vi "CLC_Gen3_L1_eleGainPhase_ENA.vi"() -> ()   [LabVIEW 2023, in "Clover_Cell.lvlib"]
uses:
  lib/CTL/Keysight_VNA.ctl
  Clover_Cell.lvlib
  lib/Keysight/Keysight.lvlib
panel:
  in  "Waiting Time(ms)":u32=100
  in  "sParameter":i32=21
  in  "Step_Freq(GHz)":dbl=0.5 format="%#_13g"
  in  "Stop_Freq(GHz)":dbl=31.5
  in  "Start_Freq(GHz)":dbl=26.5
  in  "Polarity":u16(ring) items=["H", "V"]
  in  "TRXmode":u16(ring)=1 items=["Rx"=2, "Tx"=1]
  out "Step-2":bool
  out "PHASE 2":i32
  out "GAIN 2":i32
  out "Channel 2":i32
  out "Step-1":bool
  out "Channel":i32
  out "GAIN":i32
  out "PHASE":i32
  out "Marker_array":dbl[](array[numeric])
  out "Phase":dbl[][](graph)
  in  "FileName_Note":string
  in  "VISA resource name":refnum<visa-resource-name>="TCPIP0::192.168.100.12::inst0::INSTR"
  out "Return State":bool
  out "output cluster":T1={"address"="192.168.100.111", "remote port or service name"=5025, "timeout ms (60000)"=10000}
  out "Gain":dbl[][](graph)
  out "error out":errorcluster
  # "CLC-Gen3-L1-eleGainPhase-Sweep-ENA"
  # "Setting"
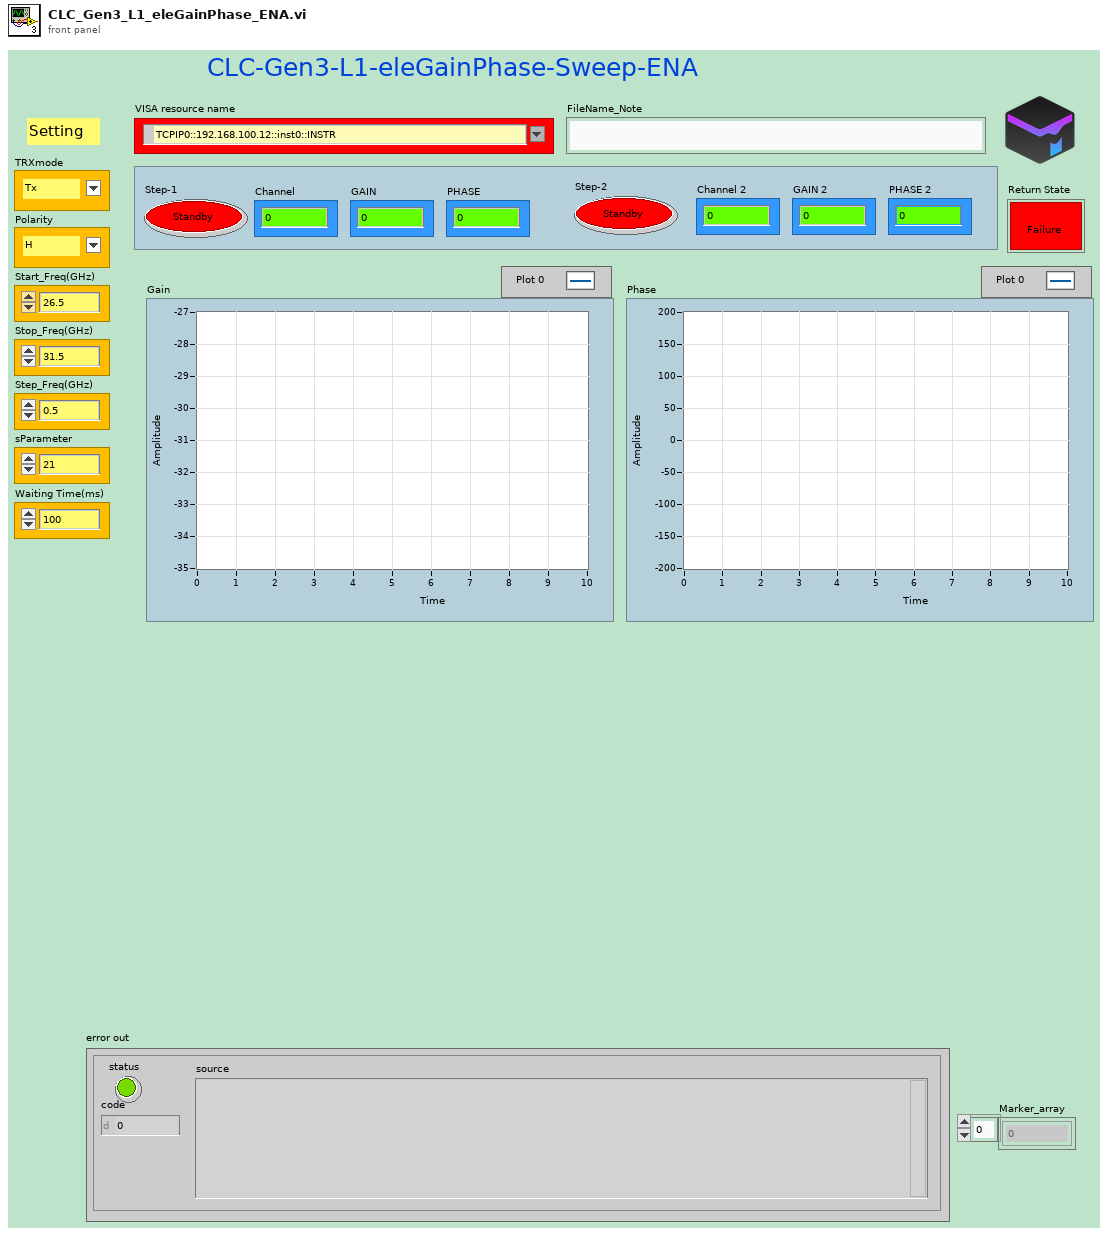
[diagram p1: front panel]
types:
  T1 = cluster{"address":string, "remote port or service name":u16, "timeout ms (60000)":i32}
  T2 = typedef "Keysight_VNA.ctl" = enum16{"Init", "queryMarker", "setSweepPoint", "setMarkerFreq", "setMeasureFormat", "setFreqStartStop", "setMarkerOnOFF", "setMarkerFormat_LOGP", "setMeasPAR_S", "setTriggerSingle", "Trigger_Save_SnP", "Trigger_Single", "Close"}
  T3 = cluster{"Mode":u16, "Polarity":u16, "CH_ON/OFF":u16, "Channel":i32, "Gain":i32, "Phase":i32}
  T4 = cluster{"setSweepPoint":i32, "Meas":i32, "Mark":i32, "Freq_GHz":dbl, "Start_Freq(GHz)":dbl, "Stop_Freq(GHz)":dbl, "sParameter":i32}
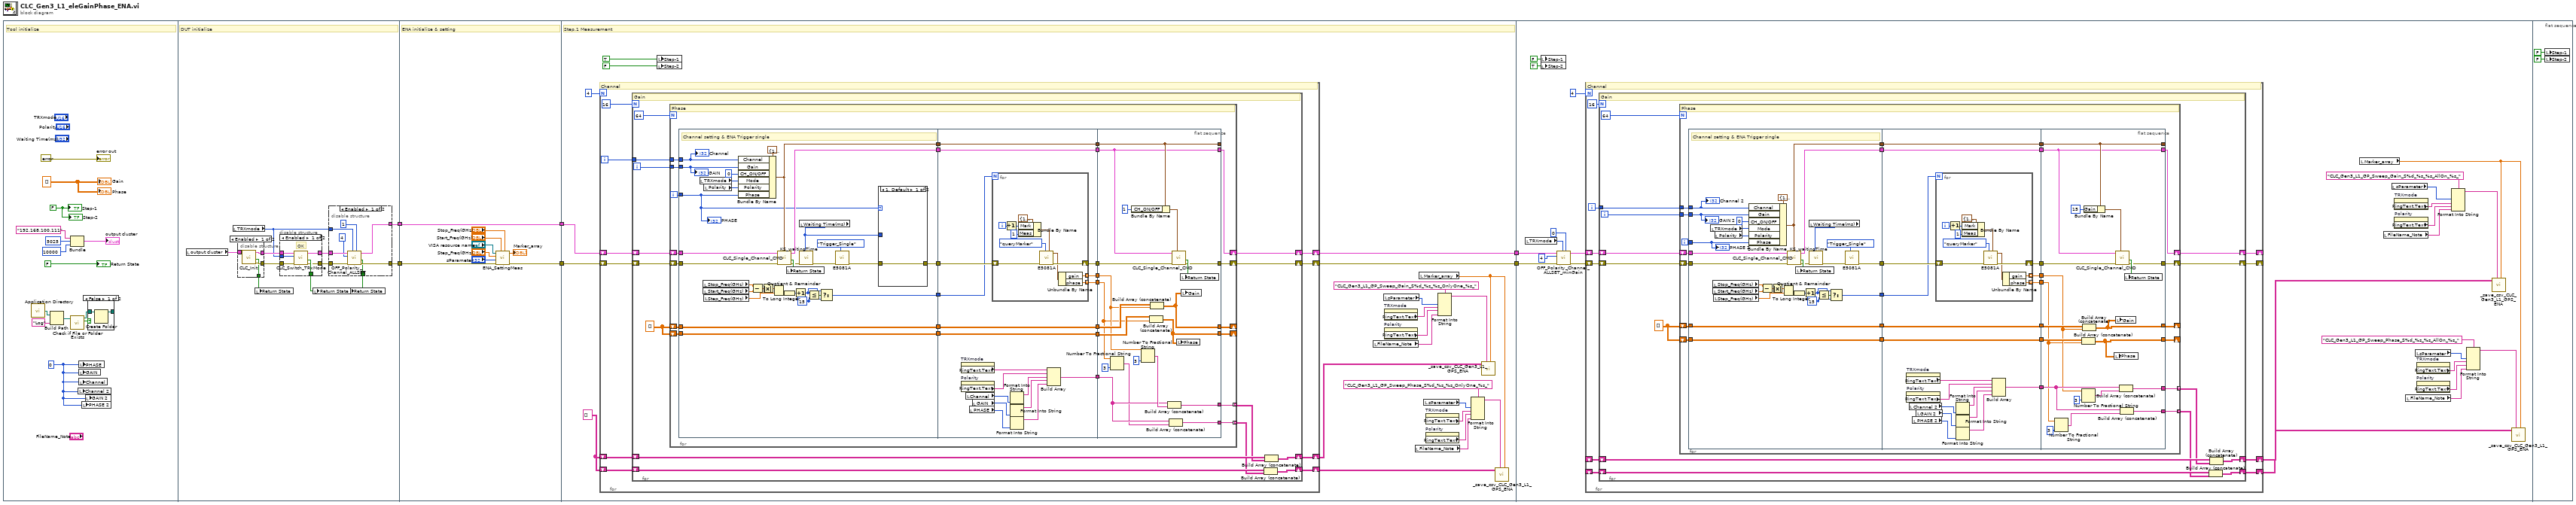
[diagram p0: block diagram]
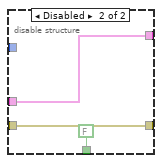
[diagram p3: hidden frame]
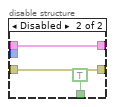
[diagram p4: hidden frame]
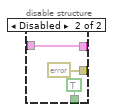
[diagram p5: hidden frame]
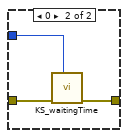
[diagram p6: hidden frame]
diagram:
  n1 = flat-sequence {
    tunnel: [w25] -> w6
    tunnel: [w29] -> w5
    tunnel: w6 -> [w70]
    tunnel: w5 -> [w63]
    tunnel: [w70] -> w4
    tunnel: [w64] -> w3
    tunnel: w4 -> [w93]
    tunnel: w3 -> [w90]
    tunnel: [w92] -> w2
    tunnel: [w91] -> w1
    tunnel: w2 -> [w249]
    tunnel: w1 -> [w250]
    frame #0 {
      w8 = FALSE ("Step-1")
      w7 = 0 ("PHASE")
      w9 = dbl[][] []
      # "Tool initialize"
      n2 = call <vilib>:"Application Directory.vi"() -> ("Application Directory"=w13:path)
      n3 = Build Path(base path=w13, name or relative path="Log") -> (appended path=w10:path)
      n4 = Bundle("address"="192.168.100.111", "remote port or service name"=u16 5025, "timeout ms (60000)"=10000) -> (→"output cluster":T1)  [unwired: 1 in]
      n5 = call <vilib>:"Check if File or Folder Exists.vi"("path"=w10) -> ("file or folder exists?"=w12:bool, "dup path"=w11:path)  [unwired: 8 in, 1 out]
      n6 = local write "Channel 2"(w7) -> ()
      n7 = local write "PHASE"(w7) -> ()
      n8 = local write "GAIN"(w7) -> ()
      n9 = local write "Channel"(w7) -> ()
      n10 = local write "PHASE 2"(w7) -> ()
      n11 = local write "GAIN 2"(w7) -> ()
      n12 = case shown="False" w12 {
        tunnel: w11 -> [w22 w23]
        tunnel: [w21 w23] -> _
        frame False {
          n13 = Create Folder(path (use dialog)=w22) -> (created path=w21:path)  [unwired: 2 in, 2 out]
        }
        frame True {
        }
      }
      "error out" <- errorcluster {"status"=FALSE, "code"=0, "source"=""} ("error out")
      "Return State" <- FALSE ("OK?")
      "Gain" <- w9
      "Phase" <- w9
      "Step-1" <- w8
      "Step-2" <- w8
    }
    frame #1 {
      # "DUT initialize"
      n14 = local read "output cluster"() -> (w34:T1)
      n15 = local read "TRXmode"() -> (w24:u16)
      n16 = disable-structure shown="Enabled" {
        disable-tunnel: w34 -> [w58 w61]
        disable-tunnel: [w57 w61] -> w33
        disable-tunnel: [w56 errorcluster {"status"=FALSE, "code"=0, "source"=""} ("error in (no error)")] -> w31
        disable-tunnel: [w55 TRUE ("OK?")] -> w26
        frame Enabled {
          n17 = call "CLC_Init.vi"("TCPIPin"=w58) -> ("error out"=w56:errorcluster, "Status"=w55:bool, "TCPIPin 2"=w57:T1)  [unwired: 8 in]
        }
        frame Disabled {
        }
      }
      n18 = local write "Return State"(w26) -> ()
      n19 = disable-structure shown="Enabled" {
        disable-tunnel: w33 -> [w51 w53]
        disable-tunnel: [w50 TRUE ("OK?")] -> w32
        disable-tunnel: w31 -> [w49 w52]
        disable-tunnel: [w48 w52] -> w30
        disable-tunnel: [w47 w53] -> w28
        disable-tunnel: w24 -> [w46 _]
        frame Enabled {
          # "OK"
          n20 = call "CLC_Switch_TRxMode.vi"("error in (no error)"=w49, "Text Ring"=w46, "TCPIPin"=w51) -> ("error out"=w48:errorcluster, "OK?"=w50:bool, "TCPIPin 2"=w47:T1)  [unwired: 6 in]
        }
        frame Disabled {
        }
      }
      n21 = local write "Return State"(w32) -> ()
      n22 = disable-structure shown="Enabled" {
        disable-tunnel: w30 -> [w42 w44]
        disable-tunnel: [w41 w44] -> w29
        disable-tunnel: w28 -> [w40 w43]
        disable-tunnel: [w39 FALSE ("OK?")] -> w27
        disable-tunnel: w24 -> [w37 _]
        disable-tunnel: [w35 w43] -> w25
        frame Enabled {
          n23 = call "OFF_Polarity_Channel_ALLSET.vi"("CH_ON:0/OFF:1"=u16 1, "Mode"=w37, "error in"=w42, "Channel"=4, "TCPIPin"=w40) -> ("error out"=w41:errorcluster, "OK?"=w39:bool, "TCPIPout"=w35:T1)  [unwired: 4 in]
        }
        frame Disabled {
        }
      }
      n24 = local write "Return State"(w27) -> ()
    }
    frame #2 {
      # "ENA initialize & setting"
      n25 = call "ENA_SettingMeas.vi"("Stop_Freq(GHz)"="Stop_Freq(GHz)", "Start_Freq(GHz)"="Start_Freq(GHz)", "error in"=w63, "sParameter"="sParameter", "Step_Freq(GHz)"="Step_Freq(GHz)", "VISA IN"="VISA resource name") -> ("error out"=w64:errorcluster, "Marker_array"=→"Marker_array":dbl[])  [unwired: 4 in]
    }
    frame #3 {
      w88 = string[][] []
      # "Step.1 Measurement"
      n26 = for {
        N: 4 -> [_]
        shift-right: [w102] -> w92
        shift-left: w93 -> [w103]
        shift-right: [w101] -> w91
        shift-left: w90 -> [w100]
        shift-right: [w95] -> w87
        shift-left: w88 -> [w97]
        shift-right: [w94] -> w86
        shift-left: w88 -> [w96]
        i -> [w98]
        # "Channel"
        n27 = for {
          N: 16 -> [_]
          shift-right: [w116] -> w102
          shift-left: w103 -> [w117]
          shift-right: [w115] -> w101
          shift-left: w100 -> [w114]
          tunnel: w98 -> [w112]
          shift-right: [w106] -> w95
          shift-left: w97 -> [w110]
          shift-right: [w105] -> w94
          shift-left: w96 -> [w109]
          i -> [w111]
          w104 = dbl[][] []
          # "Gain"
          n28 = for {
            N: 64 -> [_]
            shift-right: [w132] -> w116
            shift-left: w117 -> [w144]
            shift-right: [w131] -> w115
            shift-left: w114 -> [w143]
            tunnel: w112 -> [w142]
            tunnel: w111 -> [w141]
            tunnel: [w127] -> w108 mode=indexing
            tunnel: [w126] -> w107 mode=indexing
            shift-right: [w119] -> _
            shift-left: w104 -> [w123]
            shift-right: [w118] -> _
            shift-left: w104 -> [w120]
            i -> [w140]
            # "Phase"
            n29 = flat-sequence {
              tunnel: w144 -> [w173]
              tunnel: w143 -> [w172]
              tunnel: w142 -> [w171]
              tunnel: w141 -> [w168]
              tunnel: w140 -> [w145]
              tunnel: [w147] -> w139
              tunnel: [w153] -> w138
              tunnel: [w152] -> w137
              tunnel: [w151] -> w136
              tunnel: [w150] -> w124
              tunnel: w123 -> [w150]
              tunnel: [w149] -> w121
              tunnel: w120 -> [w149]
              tunnel: w139 -> [w196]
              tunnel: w138 -> [w195]
              tunnel: w137 -> [w194]
              tunnel: w136 -> [w193]
              tunnel: [w197] -> w135
              tunnel: [w195] -> w134
              tunnel: [w194] -> w133
              tunnel: [w192] -> w130
              tunnel: [w191] -> w129
              tunnel: [w182] -> w128
              tunnel: [w181] -> w125
              tunnel: w124 -> [w181]
              tunnel: [w180] -> w122
              tunnel: w121 -> [w180]
              tunnel: [w225] -> _
              tunnel: [w222] -> w132
              tunnel: [w227] -> w131
              tunnel: w135 -> [w226]
              tunnel: w134 -> [w222]
              tunnel: w133 -> [w225]
              tunnel: w130 -> [w212]
              tunnel: w129 -> [w211]
              tunnel: w128 -> [w218]
              tunnel: [w216] -> w127
              tunnel: [w215] -> w126
              tunnel: w125 -> [w214]
              tunnel: w122 -> [w213]
              tunnel: [w210] -> w119
              tunnel: [w209] -> w118
              frame #0 {
                w163 = 15 ("y")
                # "Channel setting & ENA Trigger single"
                n30 = local read "TRXmode"() -> (w169:u16)
                n31 = local read "Stop_Freq(GHz)"() -> (w156:dbl)
                n32 = local read "Start_Freq(GHz)"() -> (w155:dbl)
                n33 = local read "Step_Freq(GHz)"() -> (w154:dbl)
                n34 = local read "Polarity"() -> (w170:u16)
                n35 = Bundle By Name(cluster=T3 {"Mode"=1, "Polarity"=1, "CH_ON/OFF"=1, "Channel"=0, "Gain"=0, "Phase"=0} ("Channel params"), "Channel"=w171, "Gain"=w168, "CH_ON/OFF"=u16 0, "Mode"=w169, "Polarity"=w170, "Phase"=w145) -> (w152:T3)
                n36 = Subtract(x=w156, y=w155) -> (x-y=w162:dbl)
                n37 = Absolute Value(x=w162) -> (abs(x)=w161:dbl)
                n38 = Quotient & Remainder(x=w161, y=w154) -> (floor(x/y)=w160:dbl)  [unwired: 1 out]
                n39 = call "CLC_Single_Channel_CMD.vi"("Channel params"=w152, "error in"=w172, "TCPIPin"=w173) -> ("error out"=w167:errorcluster, "OK?"=w174:bool, "TCPIPout"=w153:T1)  [unwired: 6 in]
                n40 = To Long Integer(number=w160) -> (32bit integer=w159:i32)
                n41 = local write "Return State"(w174) -> ()
                n42 = Increment(x=w159) -> (x+1=w157:i32)
                n43 = local read "Waiting Time(ms)"() -> (w146:u32)
                n44 = call "KS_waitingTime.vi"("Waiting Time(ms)"=w146, "error in"=w167) -> ("error out"=w165:errorcluster)  [unwired: 9 in]
                n45 = Less Or Equal?(x=w157, y=w163) -> (x <= y?=w158:bool)
                n46 = Select(t=w157, s=w158, f=w163) -> (s? t:f=w151:i32)
                n47 = call "E5081A.vi"("Function_VNA"=Keysight_VNA."Trigger_Single", "error in"=w165) -> ("error out"=w148:errorcluster)  [unwired: 8 in, 1 out]
                n48 = case shown="1, Default" w145 {
                  tunnel: w148 -> [w176 w179]
                  tunnel: [w176 w178] -> w147
                  tunnel: w146 -> [_ w177]
                  frame 1, Default {
                  }
                  frame 0 {
                    n49 = call "KS_waitingTime.vi"("Waiting Time(ms)"=w177, "error in"=w179) -> ("error out"=w178:errorcluster)  [unwired: 9 in]
                  }
                }
                "PHASE" <- w145
                "GAIN" <- w168
                "Channel" <- w171
              }
              frame #1 {
                n50 = property on="TRXmode" class="Ring (strict)"() -> ("RingText.Text"=w187:string)  [unwired: 2 in, 2 out]
                n51 = property on="Polarity" class="Ring (strict)"() -> ("RingText.Text"=w186:string)  [unwired: 2 in, 2 out]
                n52 = local read "Channel"() -> (w190:i32)
                n53 = local read "PHASE"() -> (w188:i32)
                n54 = local read "GAIN"() -> (w189:i32)
                n55 = for {
                  N: w193 -> [_]
                  shift-right: [w207] -> w197
                  shift-left: w196 -> [w208]
                  tunnel: [w199] -> w192 mode=indexing
                  tunnel: [w198] -> w191 mode=indexing
                  i -> [w204]
                  n56 = Increment(x=w204) -> (x+1=w202:i32)
                  n57 = Bundle By Name(cluster=T4 {"setSweepPoint"=11, "Meas"=1, "Mark"=0, "Freq_GHz"=0.0, "Start_Freq(GHz)"=0.0, "Stop_Freq(GHz)"=0.0, "sParameter"=1} ("Input"), "Mark"=w202, "Meas"=1) -> (w201:T4)
                  n58 = call "E5081A.vi"("Input"=w201, "Function_VNA"=Keysight_VNA."queryMarker", "error in"=w208) -> ("error out"=w207:errorcluster, "queryMarker"=w200:cluster{"gain":dbl, "phase":dbl})  [unwired: 7 in]
                  n59 = Unbundle By Name(w200) -> ("gain"=w199:dbl, "phase"=w198:dbl)
                }
                n60 = Format Into String(w190) -> (resulting string=w185:string)  [unwired: 3 in, 1 out]
                n61 = Format Into String(w189) -> (resulting string=w184:string)  [unwired: 3 in, 1 out]
                n62 = Format Into String(w188) -> (resulting string=w183:string)  [unwired: 3 in, 1 out]
                n63 = Build Array(w187, w186, w185, w184, w183) -> (w182:string[])
              }
              frame #2 {
                n64 = Number To Fractional String(number=w211, precision (6)=i16 3) -> (F-format string=w217:string[])  [unwired: 2 in]
                n65 = Bundle By Name(cluster=w225, "CH_ON/OFF"=u16 1) -> (w223:T3)
                n66 = Number To Fractional String(number=w212, precision (6)=i16 3) -> (F-format string=w219:string[])  [unwired: 2 in]
                n67 = Build Array (concatenate)(w213, w211) -> (w209:dbl[][])
                n68 = Build Array (concatenate)(w214, w212) -> (w210:dbl[][])
                n69 = Build Array (concatenate)(w218, w219) -> (w216:string[])
                n70 = Build Array (concatenate)(w218, w217) -> (w215:string[])
                n71 = call "CLC_Single_Channel_CMD.vi"("Channel params"=w223, "error in"=w226, "TCPIPin"=w222) -> ("error out"=w227:errorcluster, "OK?"=w228:bool)  [unwired: 6 in, 1 out]
                n72 = local write "Phase"(w209) -> ()
                n73 = local write "Return State"(w228) -> ()
                n74 = local write "Gain"(w210) -> ()
              }
            }
          }
          n75 = Build Array (concatenate)(w109, w107) -> (w105:string[][])
          n76 = Build Array (concatenate)(w110, w108) -> (w106:string[][])
        }
      }
      n77 = local write "Step-1"(TRUE ("Step-1")) -> ()
      n78 = local write "Step-2"(FALSE ("Step-2")) -> ()
      n79 = local read "FileName_Note"() -> (w74:string)
      n80 = local read "sParameter"() -> (w77:i32)
      n81 = property on="TRXmode" class="Ring (strict)"() -> ("RingText.Text"=w76:string)  [unwired: 2 in, 2 out]
      n82 = property on="Polarity" class="Ring (strict)"() -> ("RingText.Text"=w75:string)  [unwired: 2 in, 2 out]
      n83 = local read "FileName_Note"() -> (w71:string)
      n84 = local read "Marker_array"() -> (w85:dbl[])
      n85 = local read "sParameter"() -> (w82:i32)
      n86 = property on="TRXmode" class="Ring (strict)"() -> ("RingText.Text"=w73:string)  [unwired: 2 in, 2 out]
      n87 = property on="Polarity" class="Ring (strict)"() -> ("RingText.Text"=w72:string)  [unwired: 2 in, 2 out]
      n88 = Format Into String(format string="CLC_Gen3_L1_GP_Sweep_Gain_S%d_%s_%s_OnlyOne_%s_" ("NoteName"), w77, w76, w75, w74) -> (resulting string=w83:string)  [unwired: 2 in, 1 out]
      n89 = Format Into String(format string="CLC_Gen3_L1_GP_Sweep_Phase_S%d_%s_%s_OnlyOne_%s_" ("NoteName"), w82, w73, w72, w71) -> (resulting string=w80:string)  [unwired: 2 in, 1 out]
      n90 = call "_save_csv_CLC_Gen3_L1_GPS_ENA.vi"("Marker_array"=w85, "NoteName"=w83, "array in"=w87) -> ()  [unwired: 8 in, 1 out]
      n91 = call "_save_csv_CLC_Gen3_L1_GPS_ENA.vi"("Marker_array"=w85, "NoteName"=w80, "array in"=w86) -> ()  [unwired: 8 in, 1 out]
    }
    frame #4 {
      n92 = local read "TRXmode"() -> (w247:u16)
      n93 = local write "Step-1"(FALSE ("Step-1")) -> ()
      n94 = local write "Step-2"(TRUE ("Step-2")) -> ()
      n95 = call "OFF_Polarity_Channel_ALLSET_minGain.vi"("CH_ON:0/OFF:1"=u16 0, "Mode"=w247, "error in"=w250, "Channel"=4, "TCPIPin"=w249) -> ("error out"=w251:errorcluster, "TCPIPout"=w252:T1)  [unwired: 4 in, 1 out]
      n96 = for {
        N: 4 -> [_]
        shift-right: [w262] -> _
        shift-left: w252 -> [w263]
        shift-right: [w261] -> _
        shift-left: w251 -> [w260]
        shift-right: [w255] -> w239
        shift-left: _ -> [w257]
        shift-right: [w254] -> w238
        shift-left: _ -> [w256]
        i -> [w258]
        # "Channel"
        n97 = for {
          N: 16 -> [_]
          shift-right: [w276] -> w262
          shift-left: w263 -> [w277]
          shift-right: [w275] -> w261
          shift-left: w260 -> [w274]
          tunnel: w258 -> [w272]
          shift-right: [w266] -> w255
          shift-left: w257 -> [w270]
          shift-right: [w265] -> w254
          shift-left: w256 -> [w269]
          i -> [w271]
          w264 = dbl[][] []
          # "Gain"
          n98 = for {
            N: 64 -> [_]
            shift-right: [w292] -> w276
            shift-left: w277 -> [w304]
            shift-right: [w291] -> w275
            shift-left: w274 -> [w303]
            tunnel: w272 -> [w302]
            tunnel: w271 -> [w301]
            tunnel: [w287] -> w268 mode=indexing
            tunnel: [w286] -> w267 mode=indexing
            shift-right: [w279] -> _
            shift-left: w264 -> [w283]
            shift-right: [w278] -> _
            shift-left: w264 -> [w280]
            i -> [w300]
            # "Phase"
            n99 = flat-sequence {
              tunnel: w304 -> [w332]
              tunnel: w303 -> [w331]
              tunnel: w302 -> [w330]
              tunnel: w301 -> [w327]
              tunnel: w300 -> [w321]
              tunnel: [w323] -> w299
              tunnel: [w310] -> w298
              tunnel: [w309] -> w297
              tunnel: [w308] -> w296
              tunnel: [w306] -> w284
              tunnel: w283 -> [w306]
              tunnel: [w305] -> w281
              tunnel: w280 -> [w305]
              tunnel: w299 -> [w351]
              tunnel: w298 -> [w350]
              tunnel: w297 -> [w349]
              tunnel: w296 -> [w348]
              tunnel: [w352] -> w295
              tunnel: [w350] -> w294
              tunnel: [w349] -> w293
              tunnel: [w347] -> w290
              tunnel: [w346] -> w289
              tunnel: [w337] -> w288
              tunnel: [w336] -> w285
              tunnel: w284 -> [w336]
              tunnel: [w335] -> w282
              tunnel: w281 -> [w335]
              tunnel: [w380] -> _
              tunnel: [w378] -> w292
              tunnel: [w382] -> w291
              tunnel: w295 -> [w381]
              tunnel: w294 -> [w378]
              tunnel: w293 -> [w380]
              tunnel: w290 -> [w367]
              tunnel: w289 -> [w364]
              tunnel: w288 -> [w374]
              tunnel: [w372] -> w287
              tunnel: [w371] -> w286
              tunnel: w285 -> [w369]
              tunnel: w282 -> [w368]
              tunnel: [w366] -> w279
              tunnel: [w365] -> w278
              frame #0 {
                w320 = 15 ("y")
                # "Channel setting & ENA Trigger single"
                n100 = local read "TRXmode"() -> (w328:u16)
                n101 = local read "Stop_Freq(GHz)"() -> (w313:dbl)
                n102 = local read "Start_Freq(GHz)"() -> (w312:dbl)
                n103 = local read "Step_Freq(GHz)"() -> (w311:dbl)
                n104 = local read "Polarity"() -> (w329:u16)
                n105 = Bundle By Name(cluster=T3 {"Mode"=1, "Polarity"=1, "CH_ON/OFF"=1, "Channel"=0, "Gain"=0, "Phase"=0} ("Channel params"), "Channel"=w330, "Gain"=w327, "CH_ON/OFF"=u16 0, "Mode"=w328, "Polarity"=w329, "Phase"=w321) -> (w309:T3)
                n106 = Subtract(x=w313, y=w312) -> (x-y=w319:dbl)
                n107 = Absolute Value(x=w319) -> (abs(x)=w318:dbl)
                n108 = Quotient & Remainder(x=w318, y=w311) -> (floor(x/y)=w317:dbl)  [unwired: 1 out]
                n109 = call "CLC_Single_Channel_CMD.vi"("Channel params"=w309, "error in"=w331, "TCPIPin"=w332) -> ("error out"=w326:errorcluster, "OK?"=w333:bool, "TCPIPout"=w310:T1)  [unwired: 6 in]
                n110 = To Long Integer(number=w317) -> (32bit integer=w316:i32)
                n111 = local write "Return State"(w333) -> ()
                n112 = Increment(x=w316) -> (x+1=w314:i32)
                n113 = local read "Waiting Time(ms)"() -> (w307:u32)
                n114 = call "KS_waitingTime.vi"("Waiting Time(ms)"=w307, "error in"=w326) -> ("error out"=w324:errorcluster)  [unwired: 9 in]
                n115 = Less Or Equal?(x=w314, y=w320) -> (x <= y?=w315:bool)
                n116 = Select(t=w314, s=w315, f=w320) -> (s? t:f=w308:i32)
                n117 = call "E5081A.vi"("Function_VNA"=Keysight_VNA."Trigger_Single", "error in"=w324) -> ("error out"=w323:errorcluster)  [unwired: 8 in, 1 out]
                "PHASE 2" <- w321
                "GAIN 2" <- w327
                "Channel 2" <- w330
              }
              frame #1 {
                n118 = property on="TRXmode" class="Ring (strict)"() -> ("RingText.Text"=w342:string)  [unwired: 2 in, 2 out]
                n119 = property on="Polarity" class="Ring (strict)"() -> ("RingText.Text"=w341:string)  [unwired: 2 in, 2 out]
                n120 = local read "Channel 2"() -> (w345:i32)
                n121 = local read "PHASE 2"() -> (w343:i32)
                n122 = local read "GAIN 2"() -> (w344:i32)
                n123 = for {
                  N: w348 -> [_]
                  shift-right: [w362] -> w352
                  shift-left: w351 -> [w363]
                  tunnel: [w354] -> w347 mode=indexing
                  tunnel: [w353] -> w346 mode=indexing
                  i -> [w359]
                  n124 = Increment(x=w359) -> (x+1=w357:i32)
                  n125 = Bundle By Name(cluster=T4 {"setSweepPoint"=11, "Meas"=1, "Mark"=0, "Freq_GHz"=0.0, "Start_Freq(GHz)"=0.0, "Stop_Freq(GHz)"=0.0, "sParameter"=1} ("Input"), "Mark"=w357, "Meas"=1) -> (w356:T4)
                  n126 = call "E5081A.vi"("Input"=w356, "Function_VNA"=Keysight_VNA."queryMarker", "error in"=w363) -> ("error out"=w362:errorcluster, "queryMarker"=w355:cluster{"gain":dbl, "phase":dbl})  [unwired: 7 in]
                  n127 = Unbundle By Name(w355) -> ("gain"=w354:dbl, "phase"=w353:dbl)
                }
                n128 = Format Into String(w345) -> (resulting string=w340:string)  [unwired: 3 in, 1 out]
                n129 = Format Into String(w344) -> (resulting string=w339:string)  [unwired: 3 in, 1 out]
                n130 = Format Into String(w343) -> (resulting string=w338:string)  [unwired: 3 in, 1 out]
                n131 = Build Array(w342, w341, w340, w339, w338) -> (w337:string[])
              }
              frame #2 {
                n132 = Number To Fractional String(number=w364, precision (6)=i16 3) -> (F-format string=w373:string[])  [unwired: 2 in]
                n133 = Build Array (concatenate)(w368, w364) -> (w365:dbl[][])
                n134 = Number To Fractional String(number=w367, precision (6)=i16 3) -> (F-format string=w375:string[])  [unwired: 2 in]
                n135 = Build Array (concatenate)(w369, w367) -> (w366:dbl[][])
                n136 = Bundle By Name(cluster=w380, "Gain"=15) -> (w379:T3)
                n137 = local write "Phase"(w365) -> ()
                n138 = call "CLC_Single_Channel_CMD.vi"("Channel params"=w379, "error in"=w381, "TCPIPin"=w378) -> ("error out"=w382:errorcluster, "OK?"=w383:bool)  [unwired: 6 in, 1 out]
                n139 = local write "Gain"(w366) -> ()
                n140 = Build Array (concatenate)(w374, w375) -> (w372:string[])
                n141 = Build Array (concatenate)(w374, w373) -> (w371:string[])
                n142 = local write "Return State"(w383) -> ()
              }
            }
          }
          n143 = Build Array (concatenate)(w269, w267) -> (w265:string[][])
          n144 = Build Array (concatenate)(w270, w268) -> (w266:string[][])
        }
      }
      n145 = local read "Marker_array"() -> (w245:dbl[])
      n146 = local read "FileName_Note"() -> (w232:string)
      n147 = local read "sParameter"() -> (w235:i32)
      n148 = property on="TRXmode" class="Ring (strict)"() -> ("RingText.Text"=w234:string)  [unwired: 2 in, 2 out]
      n149 = property on="Polarity" class="Ring (strict)"() -> ("RingText.Text"=w233:string)  [unwired: 2 in, 2 out]
      n150 = local read "FileName_Note"() -> (w229:string)
      n151 = local read "sParameter"() -> (w243:i32)
      n152 = property on="TRXmode" class="Ring (strict)"() -> ("RingText.Text"=w231:string)  [unwired: 2 in, 2 out]
      n153 = property on="Polarity" class="Ring (strict)"() -> ("RingText.Text"=w230:string)  [unwired: 2 in, 2 out]
      n154 = Format Into String(format string="CLC_Gen3_L1_GP_Sweep_Gain_S%d_%s_%s_AllOn_%s_" ("NoteName"), w235, w234, w233, w232) -> (resulting string=w244:string)  [unwired: 2 in, 1 out]
      n155 = Format Into String(format string="CLC_Gen3_L1_GP_Sweep_Phase_S%d_%s_%s_AllOn_%s_" ("NoteName"), w243, w231, w230, w229) -> (resulting string=w242:string)  [unwired: 2 in, 1 out]
      n156 = call "_save_csv_CLC_Gen3_L1_GPS_ENA.vi"("Marker_array"=w245, "NoteName"=w244, "array in"=w239) -> ()  [unwired: 8 in, 1 out]
      n157 = call "_save_csv_CLC_Gen3_L1_GPS_ENA.vi"("Marker_array"=w245, "NoteName"=w242, "array in"=w238) -> ()  [unwired: 8 in, 1 out]
    }
    frame #5 {
      n158 = local write "Step-1"(FALSE ("Step-1")) -> ()
      n159 = local write "Step-2"(FALSE ("Step-2")) -> ()
    }
  }
